vi "Scope_5782_PID.vi"() -> ()   [LabVIEW 2013]
uses:
  <vilib>/userdefined/High Color/nirio_resource_hc.ctl
  FPGA/DataMode.ctl
  <vilib>/Analysis/4window.llb/windowTd.ctl
  Host/Scope/controls/power_spectrum_unit.ctl
  Host/Scope5782/Scope/controls/5782_trigger_type.ctl
  Host/Scope/controls/Data_calc_mode.ctl
  Host/Scope/controls/Data_display_mode.ctl
  Host/Scope/controls/Graph_references.ctl
  Host/Scope/controls/graph_controls.ctl
  Host/Scope/controls/Channel_select.ctl
  Host/Scope5782/Config/FPGAref_5782.ctl
  Host/Communication/response.ctl
  Host/Communication/driver_status.ctl
  Host/Communication/Driver/RemoteConnection/RemoteReferences.ctl
  Host/Communication/Driver/TcpServerDriver/TcpServerDriver.lvclass
  Host/Scope/controls/ScopeMode.ctl
  Host/Communication/global_stop.vi
  <vilib>/FPGAPlugInAG/PXIe-7975R/niLvFpga_Open_PXIe-7975R.vi
  <vilib>/rvi/interface/common/dynamic/niFpgaDynamicAddResources.vi
  <vilib>/rvi/interface/common/niFpgaWaitOnOcc.vi
  <vilib>/Utility/error.llb/Error Cluster From Error Code.vi
  <vilib>/rvi/errors/niLvFpgaAdjustHostInterfaceError.vi
  <vilib>/FPGAPlugInAG/Dynamic/niLvFpga_Close_Dynamic.vi
  <vilib>/rvi/interface/nirviOpenFPGA/nirviOpenFPGA.xnode
  FPGA Bitfiles/mixer_FPGATarget2_FPGAmain5782PIDt_FQeTUQzgJng.lvbitx
  <vilib>/rvi/interface/nirviReadWriteControl/nirviReadWriteControl.xnode
  <vilib>/rvi/interface/nirviCloseFPGA/nirviCloseFPGA.xnode
  Host/Utilities/Ticker/Ticker.lvclass
  NiFpgaLv.dll
  <vilib>/rvi/interface/Simulation/niFpgaSimulationCallBeginRW.vi
  Host/Communication/Driver/RemoteConnection/RemoteConnection.lvclass
  <vilib>/Analysis/NI_AALPro.lvlib
panel:
  in  "Kp":fxp<+/-,32,4>
  in  "Kd/T":fxp<+/-,32,4>
  in  "Ki*T":fxp<+/-,32,4>
  in  "Feedback":bool
  in  "b":fxp<+/-,16,2>
  in  "a":fxp<+/-,16,2>
  in  "Fequency [kHz]":dbl format="%#_8g"
  in  "#bins":i32=1 min=1 max=16
  in  "ch1 DC offset":dbl caption="DC offset\nChannel 1"
  in  "ch0 DC offset":dbl caption="DC offset\nChannel 0"
  in  "Output delay delta":dbl(slide) scale=0.0..6.0
  in  "Output delay":dbl(slide) scale=0.0..6.0
  in  "Chart length":i32=200000
  in  "Trigmode":enum32{"Triggered", "Continuous"}(radio)
  in  "Refence for phase":T1
  in  "Graph_refs":T2
  out "Lower chart":dbl[][](graph)
  out "Upper chart":dbl[][](graph)
  out "Lower graph":i16[][](graph)
  in  "Buffer":T4
  in  "Display":T5
  in  "Output mixer fequency [MHz]":dbl
  in  "Trigger":T6
  in  "Ch1 Q":bool
  in  "Ch1 I":bool
  in  "Ch0 Q":bool
  in  "Ch0 I":bool
  in  "Ch1":bool
  in  "Ch0":bool
  out "stop 2":bool
  in  "Zoom freq X":bool
  in  "Zoom freq Y":bool
  in  "Zoom time Y":bool
  in  "Zoom time X":bool
  in  "Unit":T7
  in  "Window":T8=1 items=["Rectangle"=0, "Hanning"=1, "Hamming"=2, "Blackman-Harris"=3, "Exact Blackman"=4, "Blackman"=5, "Flat Top"=6, "4 Term B-Harris "=7, "7 Term B-Harris"=8, "Low Sidelobe"=9, "Blackman Nuttall"=11, "Triangle"=30, "Bartlett-Hanning"=31, "Bohman"=32, "Parzen"=33, "Welch"=34, "Kaiser"=60, "Dolph-Chebyshev"=61, "Gaussian"=62]
  in  "Samples per 5782 record":i32
  in  "Phase offset (deg)":dbl
  in  "Fequency [MHz]":dbl format="%#_8g"
  in  "Mode":T9
  in  "Mixer freq [MHz]":dbl
  out "freqdata":cluster{"f0":dbl, "df":dbl, "magnitude":dbl[]}[](graph)
  out "Upper graph":i16[][](graph)
  in  "Rumode":bool
  in  "Singleshot":bool
  out "error IO":errorcluster
  in  "stop":bool
  in  "resource name":T10="RIO0"
  out "Clocking Option Configured?":bool
  out "Configured?":bool
  # "FPGA setup"
  # "V"
  # "V"
  # "Output delay"
  # "ns"
  # "Auto Zoom"
  # "Output delay delta"
  # "ps"
  # "5782"
  # "Amplitude modulation"
  # "Simulated data"
  # "FFT"
  # "Auto Zoom"
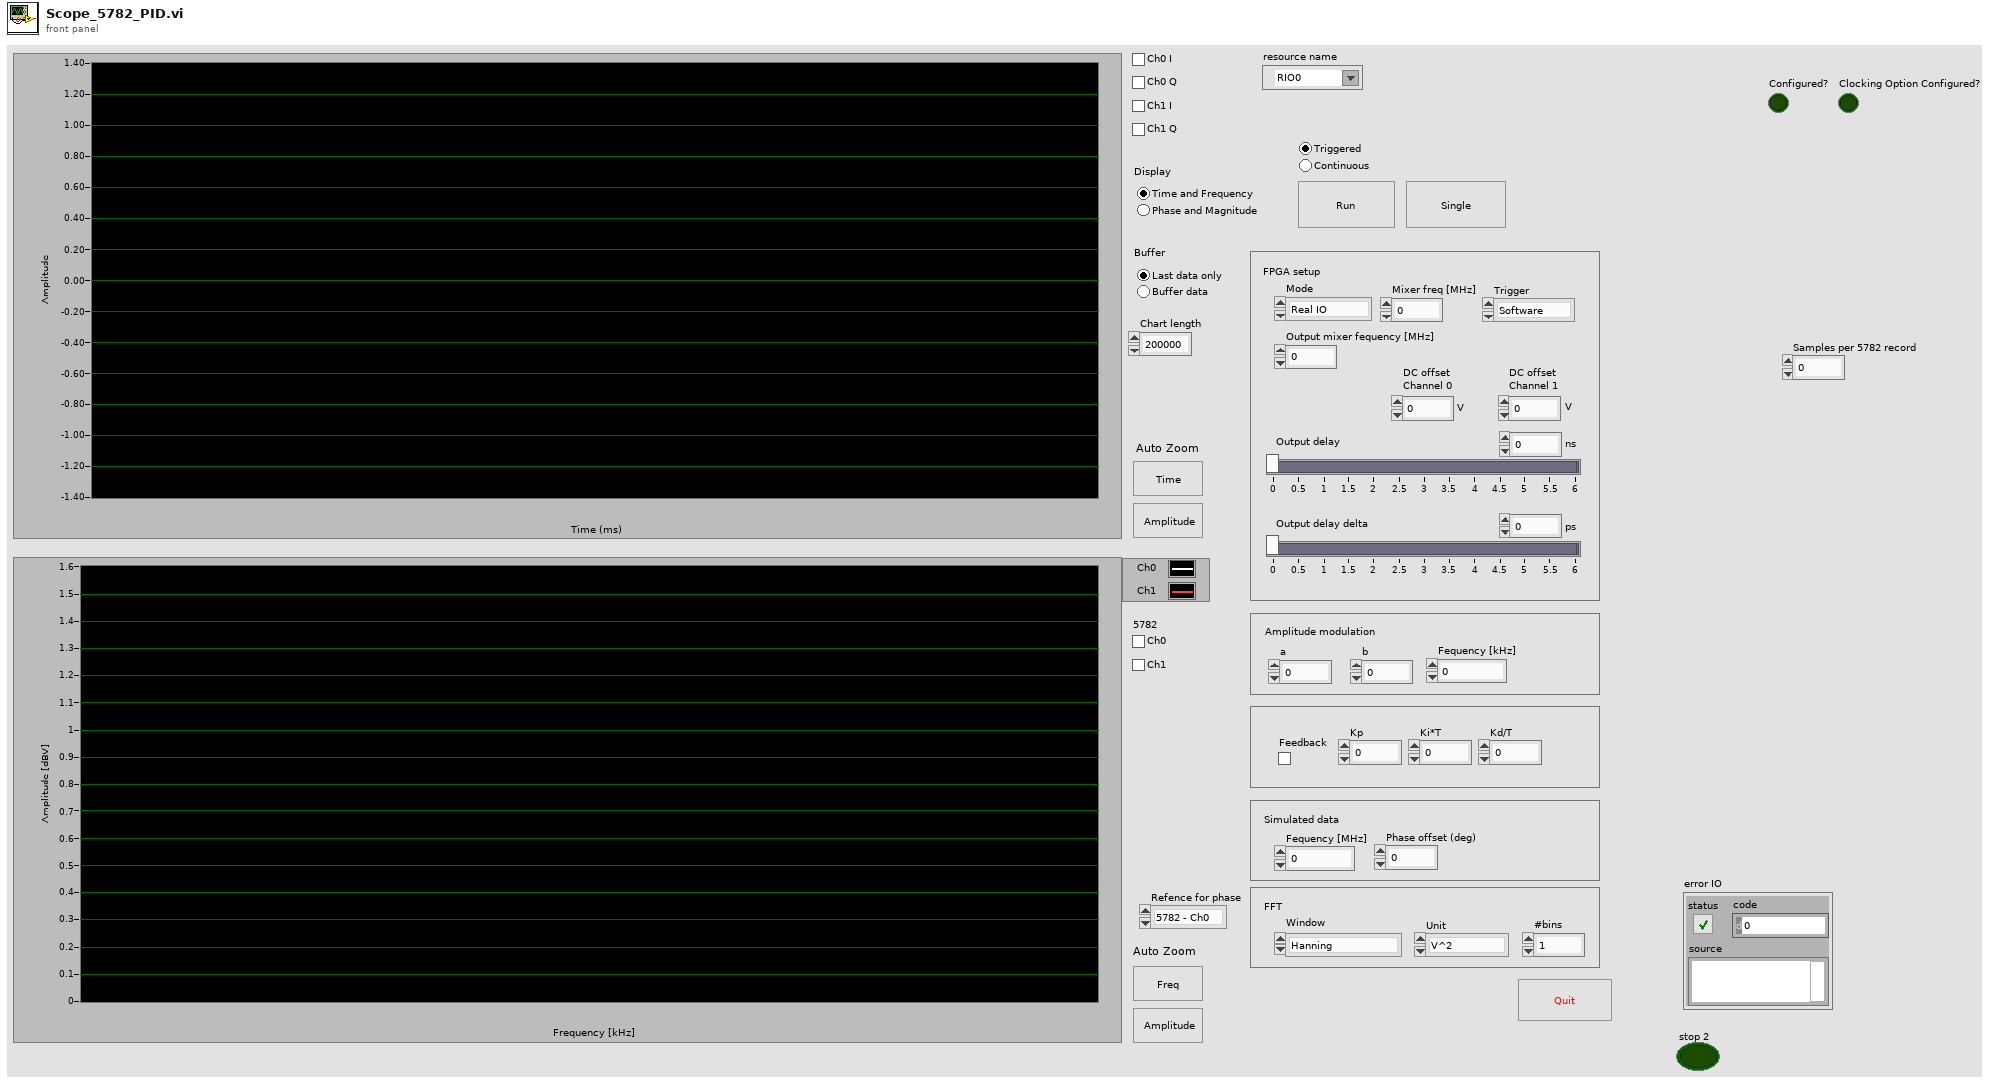
[diagram p1: front panel]
types:
  T1 = typedef "Channel_select.ctl" = enum16{"5782 - Ch0", "5782 - Ch1"}
  T2 = typedef "Graph_references.ctl" = cluster{"upper":T3, "lower":T3, "Freq graph":refnum<vi>}
  T3 = typedef "graph_controls.ctl" = cluster{"Graph":refnum<vi>, "Time btn":refnum<vi>, "Amplitude btn":refnum<vi>, "Chart":refnum<vi>}
  T4 = typedef "Data_display_mode.ctl" = enum32{"Last data only", "Buffer data"}
  T5 = typedef "Data_calc_mode.ctl" = enum32{"Time and Frequency", "Phase and Magnitude"}
  T6 = typedef "5782_trigger_type.ctl" = enum16{"Software", "Trigger input"}
  T7 = typedef "power_spectrum_unit.ctl" = enum16{"V^2", "V", "dBV"}
  T8 = typedef "NI_AALPro.lvlib/windowTd.ctl" = u32
  T9 = typedef "DataMode.ctl" = enum16{"Real IO", "Simulated"}
  T10 = typedef "nirio_resource_hc.ctl" = tag
  T11 = typedef "RemoteConnection.lvclass/RemoteReferences.ctl" = cluster{"a":refnum<vi>, "b":refnum<vi>, "fm":refnum<vi>}
  T12 = typedef "response.ctl" = cluster{"driver status":T13, "Sender":string, "Type":i32, "Variant":variant}
  T13 = typedef "driver_status.ctl" = enum16{"Normal", "Startup", "Connection lost", "Reconnected", "Timeout", "Idle", "Busy"}
  T14 = typedef "FPGAref_5782.ctl" = refnum<k20>
  T15 = enum8{"Internal Clock PLL Off", "Internal Clock PLL On (REF IN)", "External Clock (CLK_IN)", "Internal Clock PLL On (IoModSyncClk)"}
  T16 = typedef "message_queue.ctl" = refnum<queue>
  T17 = typedef "scope_params_5782.ctl" = cluster{"scope mode":T18, "ticker":refnum<class "Ticker.lvclass">, "samples per record":i32, "FPGA ref":T14, "data mode":T9, "5782 Trigger":T6, "Chart length":i32, "RemoteConnection":refnum<class "RemoteConnection.lvclass">}
  T18 = typedef "ScopeMode.ctl" = enum16{"Stopped", "Single", "Running", "Continuous"}
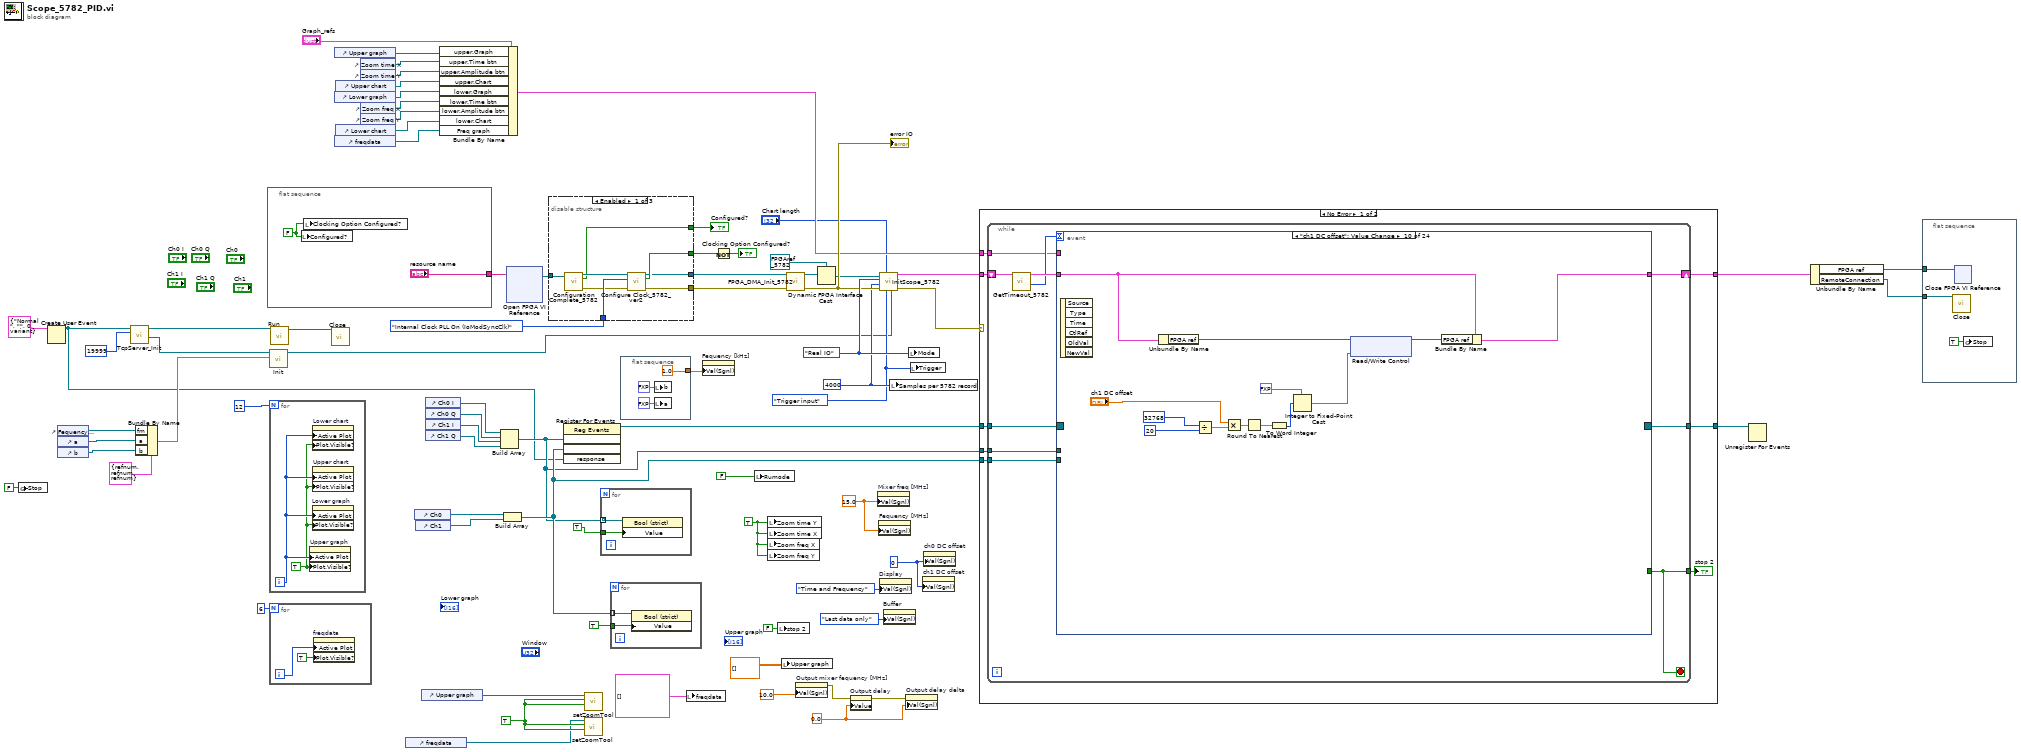
[diagram p0: block diagram]
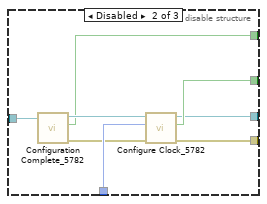
[diagram p2: hidden frame]
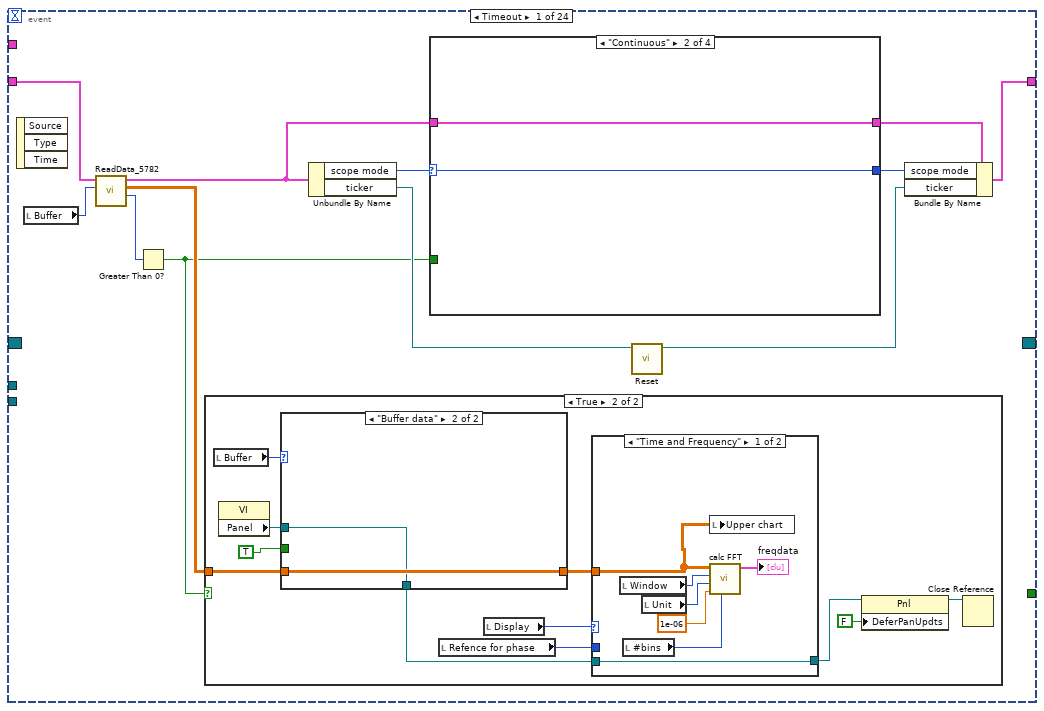
[diagram p4: hidden frame]
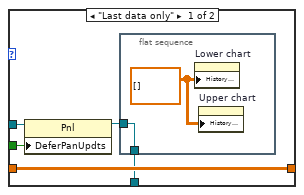
[diagram p6: hidden frame]
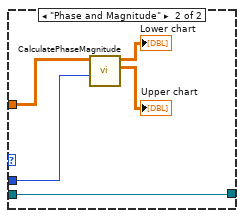
[diagram p7: hidden frame]
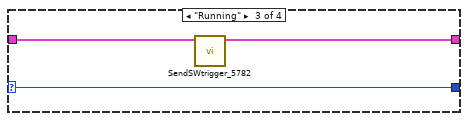
[diagram p9: hidden frame]
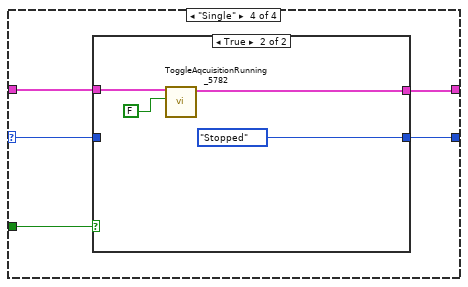
[diagram p10: hidden frame]
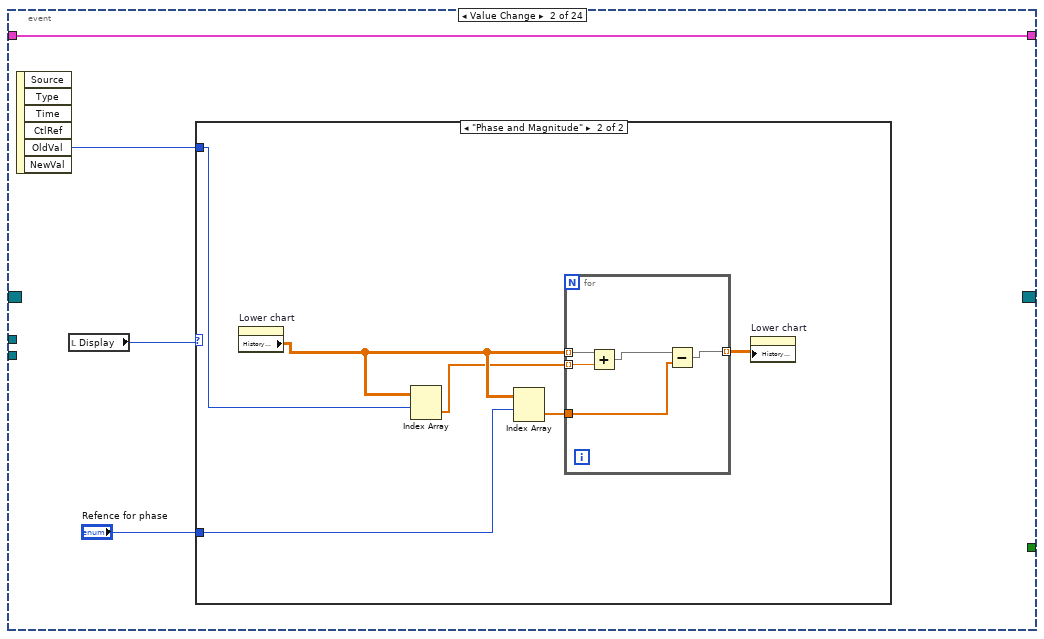
[diagram p12: hidden frame]
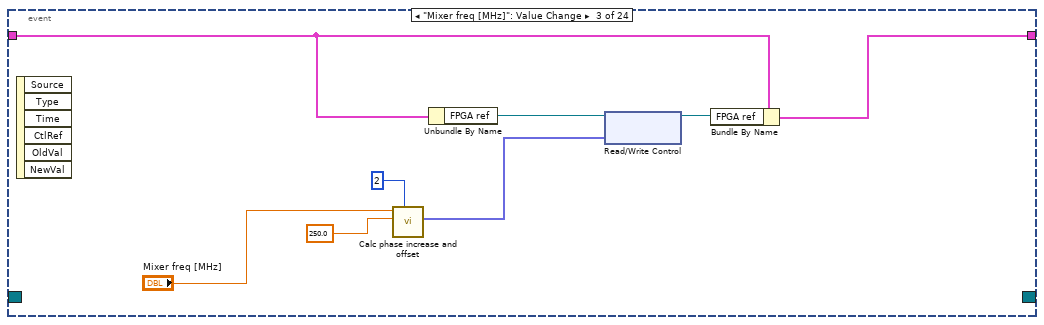
[diagram p14: hidden frame]
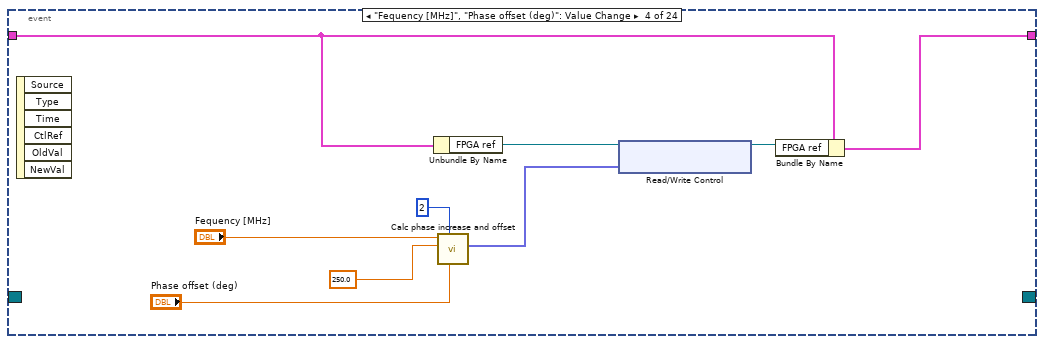
[diagram p15: hidden frame]
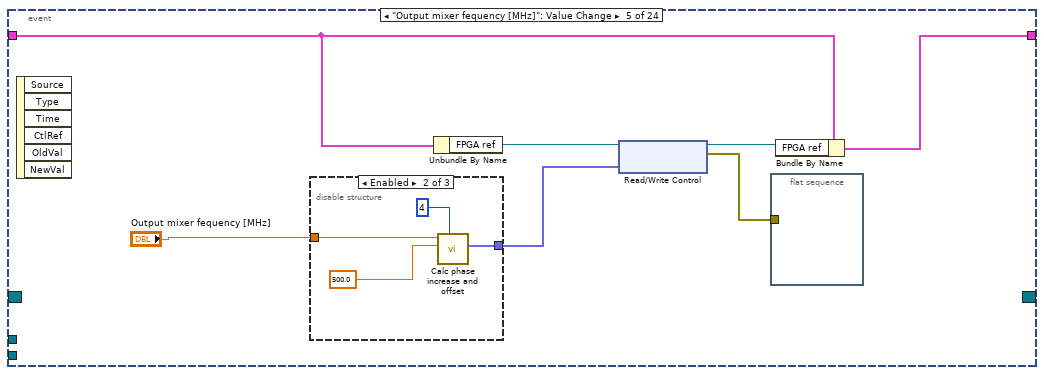
[diagram p16: hidden frame]
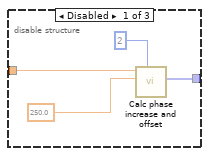
[diagram p17: hidden frame]
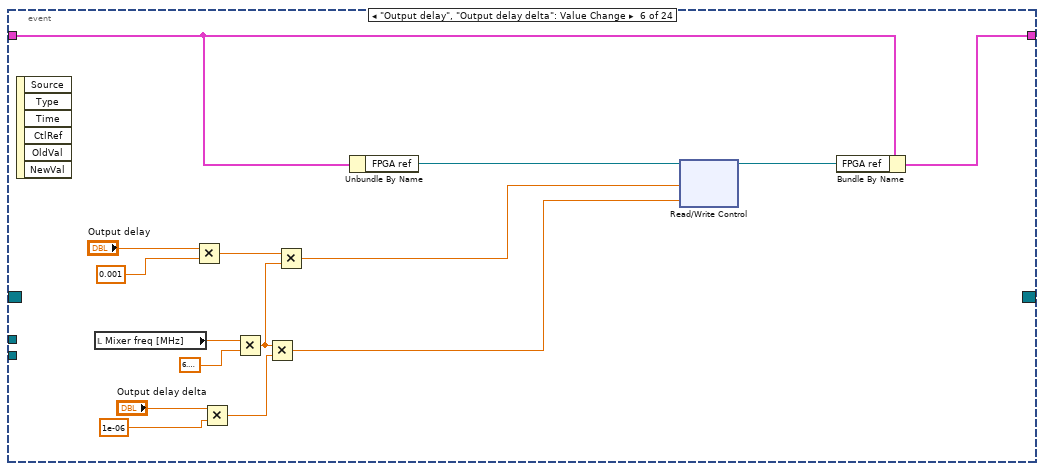
[diagram p19: hidden frame]
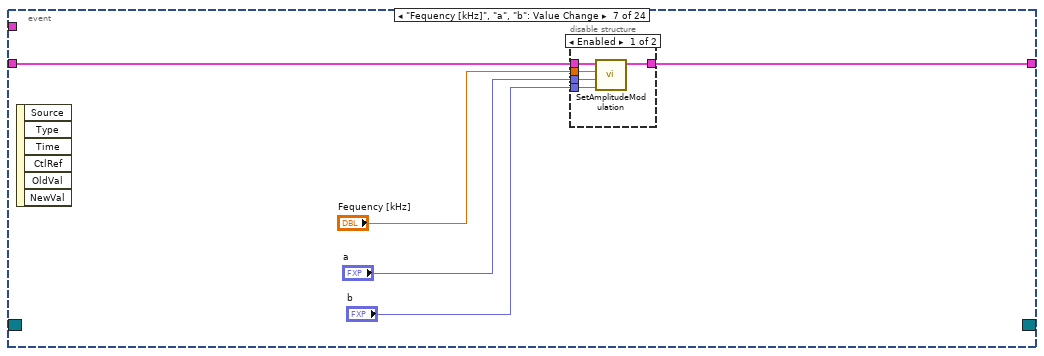
[diagram p20: hidden frame]
diagram:
  w21 = i16 0 ("Value (Signaling)")
  w22 = 0.0 ("Value (Signaling)")
  w45 = 5782_trigger_type."Trigger input" ("Trigger")
  w51 = TRUE ("Zoom  X")
  w61 = TRUE ("Rumode")
  w60 = DataMode."Real IO" ("Mode")
  w47 = 4000 ("Samples to aqcuire")
  w72 = 15.0 ("Mixer requency [MHz]")
  n1 = global write "global_stop.vi" "Stop"(FALSE ("Stop")) -> ()
  n2 = Create User Event(user event datatype=T12 {"driver status"=enum."Normal", "Sender"="", "Type"=0, "Variant"=variant} ("response")) -> (user event=w5:refnum<user-event>)  [unwired: 1 in, 1 out]
  n3 = control-ref of="Fequency [kHz]"() -> (w7:refnum<vi>)
  n4 = control-ref of="a"() -> (w8:refnum<vi>)
  n5 = control-ref of="b"() -> (w6:refnum<vi>)
  n6 = call "TcpServer_Init.vi"("local port"=u16 19999, "response event"=w5) -> ("Message queue"=w13:T16, "TcpServerDriver"=w10:refnum<class "TcpServerDriver.lvclass">)  [unwired: 8 in]
  n7 = Bundle By Name(cluster=T11 {"a"=refnum, "b"=refnum, "fm"=refnum} ("refs"), "fm"=w7, "a"=w8, "b"=w6) -> (w15:T11)
  n8 = flat-sequence {
    tunnel: ["resource name"] -> w62
    frame #0 {
      w77 = FALSE ("Trigger Acquisition")
      n9 = local write "Configured?"(w77) -> ()
      n10 = local write "Clocking Option Configured?"(w77) -> ()
    }
  }
  n11 = call "Init.vi"("refs"=w15, "server queue"=w13) -> ("RemoteConnection"=w4:refnum<class "RemoteConnection.lvclass">)  [unwired: 9 in]
  n12 = for {
    N: 12 -> [_]
    i -> [w80]
    w79 = TRUE ("Plot.Visible")
    n13 = property on="Upper graph" class="WFGraph (strict)"("Active Plot"=w80, "Plot.Visible?"=w79) -> ()  [unwired: 2 in, 2 out]
    n14 = property on="Lower graph" class="WFGraph (strict)"("Active Plot"=w80, "Plot.Visible?"=w79) -> ()  [unwired: 2 in, 2 out]
    n15 = property on="Lower chart" class="WFChart (strict)"("Active Plot"=w80, "Plot.Visible?"=w79) -> ()  [unwired: 2 in, 2 out]
    n16 = property on="Upper chart" class="WFChart (strict)"("Active Plot"=w80, "Plot.Visible?"=w79) -> ()  [unwired: 2 in, 2 out]
  }
  n17 = for {
    N: 6 -> [_]
    i -> [w81]
    n18 = property on="freqdata" class="WFGraph (strict)"("Active Plot"=w81, "Plot.Visible?"=TRUE ("Plot.Visible")) -> ()  [unwired: 2 in, 2 out]
  }
  n19 = call-dynamic "Run.vi"("BaseDriver in"=w10) -> ("BaseDriver out"=w11:refnum<class "TcpServerDriver.lvclass">)  [unwired: 9 in, 1 out]
  n20 = call-dynamic "Close.vi"("BaseDriver in"=w11) -> ()  [unwired: 9 in, 2 out]
  n21 = control-ref of="Upper graph"() -> (w42:refnum<vi>)
  n22 = control-ref of="Lower graph"() -> (w38:refnum<vi>)
  n23 = control-ref of="freqdata"() -> (w34:refnum<vi>)
  n24 = control-ref of="Upper chart"() -> (w39:refnum<vi>)
  n25 = control-ref of="Lower chart"() -> (w35:refnum<vi>)
  n26 = control-ref of="Zoom time X"() -> (w41:refnum<vi>)
  n27 = control-ref of="Zoom time Y"() -> (w40:refnum<vi>)
  n28 = control-ref of="Zoom freq X"() -> (w37:refnum<vi>)
  n29 = control-ref of="Zoom freq Y"() -> (w36:refnum<vi>)
  n30 = control-ref of="freqdata"() -> (w49:refnum<vi>)
  n31 = control-ref of="Ch0"() -> (w57:refnum<vi>)
  n32 = control-ref of="Ch1"() -> (w58:refnum<vi>)
  n33 = control-ref of="Upper graph"() -> (w50:refnum<vi>)
  n34 = control-ref of="Ch0 I"() -> (w53:refnum<vi>)
  n35 = control-ref of="Ch0 Q"() -> (w54:refnum<vi>)
  n36 = control-ref of="Ch1 I"() -> (w55:refnum<vi>)
  n37 = control-ref of="Ch1 Q"() -> (w56:refnum<vi>)
  n38 = Bundle By Name(cluster="Graph_refs", "upper.Graph"=w42, "upper.Time btn"=w41, "upper.Amplitude btn"=w40, "upper.Chart"=w39, "lower.Graph"=w38, "lower.Time btn"=w37, "lower.Amplitude btn"=w36, "lower.Chart"=w35, "Freq graph"=w34) -> (w33:T2)
  n39 = Build Array(w53, w54, w55, w56) -> (w52:refnum<vi>[])
  n40 = Build Array(w57, w58) -> (w64:refnum<vi>[])
  n41 = xnode "Open FPGA VI Reference"("resource name"=w62) -> ("FPGA VI Reference Out"=w27:refnum<k20>)  [unwired: 1 in, 1 out]
  n42 = disable-structure shown="Enabled" {
    disable-tunnel: [w90 w98 _] -> w29
    disable-tunnel: T15."Internal Clock PLL On (IoModSyncClk)" ("Clock Source") -> [w89 w97 _]
    disable-tunnel: [w87 w95 _] -> w28
    disable-tunnel: [w85 w92 w99] -> w20
    disable-tunnel: w27 -> [w83 w94 w99]
    disable-tunnel: [w84 w91 _] -> w25
    frame Enabled {
      n43 = call "Configuration Complete_5782.vi"("FPGA VI Reference in"=w83) -> ("error out"=w88:errorcluster, "Configured?"=w84:bool, "FPGA VI Reference out"=w86:refnum<k20>)  [unwired: 8 in]
      n44 = call "Configure Clock_5782_ver2.vi"("error in"=w88, "Clock Source"=w89, "FPGA VI Reference"=w86) -> ("error out"=w87:errorcluster, "Configuration Error"=w90:bool, "FPGA VI Reference out"=w85:refnum<k20>)  [unwired: 6 in]
    }
    frame Disabled {
      n45 = call "Configuration Complete_5782.vi"("FPGA VI Reference in"=w94) -> ("error out"=w96:errorcluster, "Configured?"=w91:bool, "FPGA VI Reference out"=w93:refnum<k20>)  [unwired: 8 in]
      n46 = call "Configure Clock_5782.vi"("error in"=w96, "Clock Source"=w97, "FPGA VI Reference in"=w93) -> ("error out"=w95:errorcluster, "Configuration Error"=w98:bool, "FPGA VI Reference Out"=w92:T14)  [unwired: 6 in]
    }
    frame Disabled {
    }
  }
  "Configured?" <- w25
  n47 = register-events(w52, w64, w5) -> (reference out=w68:refnum<event-registration>)  [unwired: 2 in, 1 out]
  n48 = call "setZoomTool.vi"("Zoom Y"=w51, "Zoom  X"=w51, "reference"=w49) -> ()  [unwired: 9 in]
  n49 = call "setZoomTool.vi"("Zoom Y"=w51, "Zoom  X"=w51, "reference"=w50) -> ()  [unwired: 9 in]
  n50 = for {
    tunnel: w52 -> [w101] mode=indexing
    tunnel: TRUE ("Rumode") -> [w100]
    n51 = property class="Bool (strict)"(reference=w101, "Value"=w100) -> ()  [unwired: 1 in, 2 out]
  }
  n52 = for {
    tunnel: w64 -> [w103] mode=indexing
    tunnel: TRUE ("Rumode") -> [w102]
    n53 = property class="Bool (strict)"(reference=w103, "Value"=w102) -> ()  [unwired: 1 in, 2 out]
  }
  n54 = flat-sequence {
    tunnel: [1.0 ("Value (Signaling)")] -> w19
    frame #0 {
      n55 = local write "b"(fxp<+/-,16,2> 0.0 ("b")) -> ()
      n56 = local write "a"(fxp<+/-,16,2> 1.0 ("a")) -> ()
    }
  }
  n57 = local write "freqdata"(cluster{"f0":dbl, "df":dbl, "magnitude":dbl[]}[] [] ("freqdata")) -> ()
  n58 = property on="Fequency [kHz]" class="DigNum (strict)"("Val(Sgnl)"=w19) -> ()  [unwired: 2 in, 2 out]
  n59 = Not(x=w29) -> (.not. x?=→"Clocking Option Configured?":bool)
  n60 = local write "Rumode"(FALSE ("Rumode")) -> ()
  n61 = local write "Zoom time Y"(w61) -> ()
  n62 = local write "Zoom time X"(w61) -> ()
  n63 = local write "Zoom freq X"(w61) -> ()
  n64 = local write "Zoom freq Y"(w61) -> ()
  n65 = local write "stop 2"(FALSE ("stop 2")) -> ()
  n66 = local write "Upper graph"(dbl[][] [] ("Timedata")) -> ()
  n67 = call "FPGA_DMA_Init_5782.vi"("error in (no error)"=w28, "FPGA VI Reference"=w20) -> ("error out"=w48:errorcluster, "FPGA VI Out"=w18:refnum<k20>)  [unwired: 7 in, 1 out]
  "error IO" <- w48
  n68 = property on="Output mixer fequency [MHz]" class="DigNum (strict)"("Val(Sgnl)"=10.0 ("Mixer requency [MHz]")) -> (error out=w23:errorcluster)  [unwired: 2 in, 1 out]
  n69 = Dynamic FPGA Interface Cast(Session In=T14 refnum ("FPGA ref"), Type=w18) -> (Session Out=w17:T14)
  n70 = property on="Output delay" class="Slide (strict)"(error in=w23, "Value"=w22) -> (error out=w24:errorcluster)  [unwired: 1 in, 1 out]
  n71 = property on="Mixer freq [MHz]" class="DigNum (strict)"("Val(Sgnl)"=w72) -> ()  [unwired: 2 in, 2 out]
  n72 = property on="Fequency [MHz]" class="DigNum (strict)"("Val(Sgnl)"=w72) -> ()  [unwired: 2 in, 2 out]
  n73 = call "InitScope_5782.vi"("RemoteConnection"=w4, "Trigger"=w45, "Chart length"="Chart length", "error in"=w48, "Samples Per Trigger"=w47, "data mode"=w60, "FPGA ref"=w17) -> ("error out"=w1:errorcluster, "scope params"=w76:T17)  [unwired: 3 in]
  n74 = property on="Display" class="RadioBtnsControl (strict)"("Val(Sgnl)"=Data_calc_mode."Time and Frequency" ("Value (Signaling)")) -> ()  [unwired: 2 in, 2 out]
  n75 = property on="Buffer" class="RadioBtnsControl (strict)"("Val(Sgnl)"=enum32{"Last data only", "Buffer data"}."Last data only" ("Value (Signaling)")) -> ()  [unwired: 2 in, 2 out]
  n76 = local write "Samples per 5782 record"(w47) -> ()
  n77 = property on="Output delay delta" class="Slide (strict)"(error in=w24, "Val(Sgnl)"=w22) -> ()  [unwired: 1 in, 2 out]
  n78 = local write "Mode"(w60) -> ()
  n79 = local write "Trigger"(w45) -> ()
  n80 = property on="ch1 DC offset" class="DigNum (strict)"("Val(Sgnl)"=w21) -> ()  [unwired: 2 in, 2 out]
  n81 = property on="ch0 DC offset" class="DigNum (strict)"("Val(Sgnl)"=w21) -> ()  [unwired: 2 in, 2 out]
  n82 = case shown="No Error" w1 {
    tunnel: w76 -> [w114 w397]
    tunnel: [w113 w397] -> w46
    tunnel: w68 -> [w112 w396]
    tunnel: [w111 w396] -> w67
    tunnel: w52 -> [w110 _]
    tunnel: w64 -> [w109 _]
    tunnel: w33 -> [w107 _]
    frame No Error {
      n83 = while {
        shift-right: [w124] -> w113
        shift-left: w114 -> [w123]
        tunnel: w112 -> [w120]
        tunnel: [w119] -> w111
        tunnel: w110 -> [w118]
        tunnel: w109 -> [w117]
        tunnel: [w116] -> w108
        tunnel: w107 -> [w115]
        stop <- w116 stop-if-true
        n84 = call "GetTimeout_5782.vi"("scope in"=w123) -> ("Time left"=w121:i32, "scope out"=w122:T17)  [unwired: 9 in]
        n85 = event shown="[9] \"ch1 DC offset\": Value Change" {
          selector: w120 -> [_ _ _ _ _ _ _ _ _ _ _ _ _ _ _ _ _ _ _ _ _ _ _ _]
          dyn-events: [_ _ _ _ _ _ _ _ _ _ _ _ _ _ _ _ _ _ _ _ _ _ _ _] -> w119
          timeout: w121 -> [_ _ _ _ _ _ _ _ _ _ _ _ _ _ _ _ _ _ _ _ _ _ _ _]
          tunnel: [_ _ _ _ _ _ _ _ _ _ _ _ _ _ _ _ _ _ "stop" _ _ _ _ _] -> w116
          tunnel: w122 -> [w131 w190 w208 w214 w223 w244 w253 w265 w278 w291 w297 w301 w304 w314 w322 w347 w352 w357 w360 w367 w377 w382 w388 w395]
          tunnel: [w134 w190 w206 w213 w222 w243 w252 w264 w277 w290 w296 w300 w303 w311 w319 w347 w352 w356 w360 w367 w377 w382 w388 w395] -> w124
          tunnel: w118 -> [_ _ _ _ _ _ _ _ _ _ _ _ _ _ _ w346 _ _ _ _ _ _ _ _]
          tunnel: w117 -> [_ _ _ _ _ _ _ _ _ _ _ _ _ _ _ _ w350 _ _ _ _ _ _ _]
          tunnel: w115 -> [_ _ _ _ _ _ _ _ _ _ _ _ _ _ _ _ _ _ _ _ _ _ _ w392]
          event Timeout {
            n86 = event-data() -> ()  [unwired: 1 in, 3 out]
            n87 = local read "Buffer"() -> (w125:T4)
            n88 = call "ReadData_5782.vi"("Buffer mode"=w125, "scope params"=w131) -> ("Num elements"=w127:i32, "data"=w128:dbl[][], "scope params out"=w130:T17)  [unwired: 7 in]
            n89 = Greater Than 0?(x=w127) -> (x > 0?=w126:bool)
            n90 = case shown="True" w126 {
              tunnel: w128 -> [_ w144]
              frame False {
              }
              frame True {
                n91 = local read "Buffer"() -> (w146:T4)
                n92 = property class="VI"() -> ("Panel"=w139:refnum<vi>)  [unwired: 2 in, 2 out]
                n93 = case shown="\"Buffer data\"" w146 {
                  tunnel: w144 -> [w152 w156]
                  tunnel: [w152 w156] -> w145
                  tunnel: w139 -> [w151 w155]
                  tunnel: TRUE ("Defer Panel Updates") -> [w149 _]
                  tunnel: [w148 w155] -> w137
                  frame "Last data only" {
                    n94 = property class="Pnl"(reference=w151, "DeferPanUpdts"=w149) -> (reference out=w150:refnum<vi>)  [unwired: 1 in, 1 out]
                    n95 = flat-sequence {
                      tunnel: w150 -> [w153]
                      tunnel: [w153] -> w148
                      frame #0 {
                        w154 = dbl[][] [] ("History Data")
                        n96 = property on="Lower chart" class="WFChart (strict)"("History Data"=w154) -> ()  [unwired: 2 in, 2 out]
                        n97 = property on="Upper chart" class="WFChart (strict)"("History Data"=w154) -> ()  [unwired: 2 in, 2 out]
                      }
                    }
                  }
                  frame "Buffer data" {
                  }
                }
                n98 = local read "Refence for phase"() -> (w143:T1)
                n99 = local read "Display"() -> (w147:T5)
                n100 = case shown="\"Time and Frequency\"" w147 {
                  tunnel: w145 -> [w159 w168]
                  tunnel: w143 -> [_ w165]
                  tunnel: [w158 w164] -> w141
                  tunnel: w137 -> [w158 w164]
                  frame "Time and Frequency" {
                    n101 = local read "Window"() -> (w160:T8)
                    n102 = local read "#bins"() -> (w157:i32)
                    n103 = local read "Unit"() -> (w161:T7)
                    n104 = local write "Upper chart"(w159) -> ()
                    n105 = call "calc FFT.vi"("#bins"=w157, "dt"=1e-06, "Unit"=w161, "Window"=w160, "data"=w159) -> ("Power Spectrum / PSD"=→"freqdata":cluster{"f0":dbl, "df":dbl, "magnitude":dbl[]}[])  [unwired: 6 in]
                  }
                  frame "Phase and Magnitude" {
                    n106 = call "CalculatePhaseMagnitude.vi"("phase reference channel"=w165, "data"=w168) -> ("Magnitude"=→"Upper chart":dbl[][], "Phase"=→"Lower chart":dbl[][])  [unwired: 8 in]
                  }
                }
                n107 = property class="Pnl"(reference=w141, "DeferPanUpdts"=FALSE ("Defer Panel Updates")) -> (reference out=w140:refnum<vi>)  [unwired: 1 in, 1 out]
                n108 = Close Reference(reference=w140) -> ()  [unwired: 1 in, 1 out]
              }
            }
            n109 = Unbundle By Name(w130) -> ("scope mode"=w133:T18, "ticker"=w136:refnum<class "Ticker.lvclass">)
            n110 = case shown="\"Continuous\"" w133 {
              selector: w133 -> [w170 w172 w175 w176]
              tunnel: [w170 w172 w175 w180] -> w132
              tunnel: w130 -> [w169 w171 w174 w178]
              tunnel: [w169 w171 w173 w177] -> w129
              tunnel: w126 -> [_ _ _ w179]
              frame "Stopped" {
              }
              frame "Continuous" {
              }
              frame "Running" {
                n111 = call "SendSWtrigger_5782.vi"("scope in"=w174) -> ("scope out"=w173:T17)  [unwired: 9 in, 1 out]
              }
              frame "Single" {
                n112 = case shown="True" w179 {
                  tunnel: [w181 ScopeMode."Stopped" ("scope mode")] -> w180
                  tunnel: w178 -> [w182 w185]
                  tunnel: [w182 w184] -> w177
                  tunnel: w176 -> [w181 _]
                  frame False {
                  }
                  frame True {
                    n113 = call "ToggleAqcuisitionRunning_5782.vi"("Acquisition running"=FALSE, "scope in"=w185) -> ("scope out"=w184:T17)  [unwired: 8 in, 1 out]
                  }
                }
              }
            }
            n114 = call "Reset.vi"("Ticker in"=w136) -> ("Ticker out"=w135:refnum<class "Ticker.lvclass">)  [unwired: 9 in, 1 out]
            n115 = Bundle By Name(cluster=w129, "scope mode"=w132, "ticker"=w135) -> (w134:T17)
          }
          event Value Change {
            n116 = event-data() -> ("OldVal"=w187:T1)  [unwired: 1 in, 5 out]
            n117 = local read "Display"() -> (w188:T5)
            n118 = case shown="\"Phase and Magnitude\"" w188 {
              tunnel: "Refence for phase" -> [_ w195]
              tunnel: w187 -> [_ w193]
              frame "Time and Frequency", Default {
              }
              frame "Phase and Magnitude" {
                n119 = property on="Lower chart" class="WFChart (strict)"() -> ("History Data"=w194:dbl[][])  [unwired: 2 in, 2 out]
                n120 = Index Array(array=w194, index (row)=w193) -> (element=w192:dbl[])  [unwired: 1 in]
                n121 = Index Array(array=w194, index (row)=w195) -> (element=w196:dbl[])  [unwired: 1 in]
                n122 = for {
                  tunnel: w194 -> [w199] mode=indexing
                  tunnel: w196 -> [w201]
                  tunnel: [w200] -> w191 mode=indexing
                  tunnel: w192 -> [w198] mode=indexing
                  n123 = Add(x=w199, y=w198) -> (x+y=w197:dbl[])
                  n124 = Subtract(x=w197, y=w201) -> (x-y=w200:dbl[])
                }
                n125 = property on="Lower chart" class="WFChart (strict)"("History Data"=w191) -> ()  [unwired: 2 in, 2 out]
              }
            }
          }
          event "Mixer freq [MHz]": Value Change {
            n126 = event-data() -> ()  [unwired: 1 in, 6 out]
            n127 = call "Calc phase increase and offset.vi"("# of DDS"=2, "fclk (MHz)"=250.0 ("fclk (800MHz)"), "f_generated (MHz)"="Mixer freq [MHz]") -> ("Phase out"=w202:fxp<+,64,64>[])  [unwired: 6 in, 2 out]
            n128 = Unbundle By Name(w208) -> ("FPGA ref"=w209:T14)
            n129 = xnode "Read/Write Control"("FPGA VI Reference In"=w209, "Phase 5782"=w202) -> ("FPGA VI Reference Out"=w207:T14)  [unwired: 1 in, 1 out]
            n130 = Bundle By Name(cluster=w208, "FPGA ref"=w207) -> (w206:T17)
          }
          event "Fequency [MHz]", "Phase offset (deg)": Value Change {
            n131 = event-data() -> ()  [unwired: 1 in, 6 out]
            n132 = Unbundle By Name(w214) -> ("FPGA ref"=w216:T14)
            n133 = call "Calc phase increase and offset.vi"("Phase offset (deg)"="Phase offset (deg)", "# of DDS"=2, "fclk (MHz)"=250.0 ("fclk (800MHz)"), "f_generated (MHz)"="Fequency [MHz]") -> ("Phase out"=w210:fxp<+,64,64>[])  [unwired: 5 in, 2 out]
            n134 = xnode "Read/Write Control"("FPGA VI Reference In"=w216, "Simulated phase 5782"=w210) -> ("FPGA VI Reference Out"=w215:T14)  [unwired: 1 in, 1 out]
            n135 = Bundle By Name(cluster=w214, "FPGA ref"=w215) -> (w213:T17)
          }
          event "Output mixer fequency [MHz]": Value Change {
            n136 = event-data() -> ()  [unwired: 1 in, 6 out]
            n137 = disable-structure shown="Enabled" {
              disable-tunnel: [w227 w231 _] -> w219
              disable-tunnel: "Output mixer fequency [MHz]" -> [w226 w230 _]
              frame Disabled {
                n138 = call "Calc phase increase and offset.vi"("# of DDS"=2, "fclk (MHz)"=250.0 ("fclk (800MHz)"), "f_generated (MHz)"=w226) -> ("Phase out"=w227:fxp<+,64,64>[])  [unwired: 6 in, 2 out]
              }
              frame Enabled {
                n139 = call "Calc phase increase and offset.vi"("# of DDS"=4, "fclk (MHz)"=500.0 ("fclk (800MHz)"), "f_generated (MHz)"=w230) -> ("Phase out"=w231:fxp<+,64,64>[])  [unwired: 6 in, 2 out]
              }
              frame Disabled {
              }
            }
            n140 = Unbundle By Name(w223) -> ("FPGA ref"=w225:T14)
            n141 = xnode "Read/Write Control"("FPGA VI Reference In"=w225, "Phase output"=w219) -> ("FPGA VI Reference Out"=w224:T14, "error out"=w220:errorcluster)  [unwired: 1 in]
            n142 = flat-sequence {
              tunnel: w220 -> [_]
              frame #0 {
              }
            }
            n143 = Bundle By Name(cluster=w223, "FPGA ref"=w224) -> (w222:T17)
          }
          event "Output delay", "Output delay delta": Value Change {
            n144 = event-data() -> ()  [unwired: 1 in, 6 out]
            n145 = local read "Mixer freq [MHz]"() -> (w238:dbl)
            n146 = Multiply(x="Output delay", y=0.001) -> (x*y=w239:dbl)
            n147 = Multiply(x="Output delay delta", y=1e-06) -> (x*y=w241:dbl)
            n148 = Multiply(x=w238, y=6.283185307179586) -> (x*y=w234:dbl)
            n149 = Multiply(x=w234, y=w241) -> (x*y=w235:dbl)
            n150 = Multiply(x=w239, y=w234) -> (x*y=w236:dbl)
            n151 = Unbundle By Name(w244) -> ("FPGA ref"=w248:T14)
            n152 = xnode "Read/Write Control"("FPGA VI Reference In"=w248, "Fi_start"=w236, "Fi_delta"=w235) -> ("FPGA VI Reference Out"=w247:T14)  [unwired: 1 in, 1 out]
            n153 = Bundle By Name(cluster=w244, "FPGA ref"=w247) -> (w243:T17)
          }
          event "Fequency [kHz]", "a", "b": Value Change {
            n154 = event-data() -> ()  [unwired: 1 in, 6 out]
            n155 = disable-structure shown="Enabled" {
              disable-tunnel: w253 -> [w258 w259]
              disable-tunnel: [w257 w259] -> w252
              disable-tunnel: "Fequency [kHz]" -> [w256 _]
              disable-tunnel: "a" -> [w255 _]
              disable-tunnel: "b" -> [w254 _]
              frame Enabled {
                n156 = call "SetAmplitudeModulation.vi"("b_am"=w254, "a_am"=w255, "Am freq [kHz]"=w256, "scope in"=w258) -> ("scope out"=w257:T17)  [unwired: 7 in]
              }
              frame Disabled {
              }
            }
          }
          event "Feedback": Value Change {
            n157 = event-data() -> ()  [unwired: 1 in, 6 out]
            n158 = Unbundle By Name(w265) -> ("FPGA ref"=w267:T14)
            n159 = xnode "Read/Write Control"("FPGA VI Reference In"=w267, "feedback enable"="Feedback", "Ki*Tau"="Ki*T", "Kd/Tau"="Kd/T", "Kp"="Kp") -> ("FPGA VI Reference Out"=w266:T14)  [unwired: 1 in, 1 out]
            n160 = Bundle By Name(cluster=w265, "FPGA ref"=w266) -> (w264:T17)
          }
          event "ch0 DC offset": Value Change {
            n161 = event-data() -> ()  [unwired: 1 in, 6 out]
            n162 = Unbundle By Name(w278) -> ("FPGA ref"=w280:T14)
            n163 = Divide(x=32768, y=20) -> (x/y=w274:dbl)
            n164 = Multiply(x="ch0 DC offset", y=w274) -> (x*y=w273:dbl)
            n165 = Round To Nearest(number=w273) -> (nearest integer value=w272:dbl)
            n166 = To Word Integer(number=w272) -> (16bit integer=w271:i16)
            n167 = Integer to Fixed-Point Cast(fixed-point type=fxp<+/-,16,14> 0.0 ("y"), integer=w271) -> (fixed-point=w269:fxp<+/-,16,14>)
            n168 = xnode "Read/Write Control"("FPGA VI Reference In"=w280, "DC offset chan 0"=w269) -> ("FPGA VI Reference Out"=w279:T14)  [unwired: 1 in, 1 out]
            n169 = Bundle By Name(cluster=w278, "FPGA ref"=w279) -> (w277:T17)
          }
          event "ch1 DC offset": Value Change {
            n170 = event-data() -> ()  [unwired: 1 in, 6 out]
            n171 = Unbundle By Name(w291) -> ("FPGA ref"=w293:T14)
            n172 = Divide(x=32768, y=20) -> (x/y=w287:dbl)
            n173 = Multiply(x="ch1 DC offset", y=w287) -> (x*y=w286:dbl)
            n174 = Round To Nearest(number=w286) -> (nearest integer value=w285:dbl)
            n175 = To Word Integer(number=w285) -> (16bit integer=w284:i16)
            n176 = Integer to Fixed-Point Cast(fixed-point type=fxp<+/-,16,14> 0.0 ("y"), integer=w284) -> (fixed-point=w281:fxp<+/-,16,14>)
            n177 = xnode "Read/Write Control"("FPGA VI Reference In"=w293, "DC offset chan 1"=w281) -> ("FPGA VI Reference Out"=w292:T14)  [unwired: 1 in, 1 out]
            n178 = Bundle By Name(cluster=w291, "FPGA ref"=w292) -> (w290:T17)
          }
          event Value Change {
            n179 = event-data() -> ()  [unwired: 1 in, 6 out]
            n180 = Unbundle By Name(w297) -> ("FPGA ref"=w299:T14)
            n181 = property on="Rumode" class="Bool (strict)"("Val(Sgnl)"=FALSE ("Value (Signaling)")) -> ()  [unwired: 2 in, 2 out]
            n182 = xnode "Read/Write Control"("FPGA VI Reference In"=w299, "Mode"="Mode") -> ("FPGA VI Reference Out"=w298:T14)  [unwired: 1 in, 1 out]
            n183 = Bundle By Name(cluster=w297, "FPGA ref"=w298, "data mode"="Mode") -> (w296:T17)
          }
          event Value Change {
            n184 = event-data() -> ()  [unwired: 1 in, 6 out]
            n185 = Bundle By Name(cluster=w301, "5782 Trigger"="Trigger") -> (w300:T17)
          }
          event "Samples per 5782 record": Value Change {
            n186 = event-data() -> ()  [unwired: 1 in, 6 out]
            n187 = Unbundle By Name(w304) -> ("FPGA ref"=w307:T14)
            n188 = xnode "Read/Write Control"("FPGA VI Reference In"=w307, "5782 record length"="Samples per 5782 record") -> ("FPGA VI Reference Out"=w306:T14)  [unwired: 1 in, 1 out]
            n189 = Bundle By Name(cluster=w304, "FPGA ref"=w306, "samples per record"="Samples per 5782 record") -> (w303:T17)
          }
          event "Singleshot": Value Change {
            n190 = event-data() -> ()  [unwired: 1 in, 6 out]
            n191 = local write "Rumode"(FALSE ("Rumode")) -> ()
            n192 = Bundle By Name(cluster=w314, "scope mode"=ScopeMode."Single") -> (w309:T17)
            n193 = call "ToggleContinousMode.vi"("Cont Acquisition"=FALSE, "scope in"=w309) -> ("scope out"=w308:T17)  [unwired: 8 in, 1 out]
            n194 = call "ToggleAqcuisitionRunning_5782.vi"("Acquisition running"=TRUE, "scope in"=w308) -> ("scope out"=w312:T17)  [unwired: 8 in, 1 out]
            n195 = call "SendSWtrigger_5782.vi"("scope in"=w312) -> ("scope out"=w311:T17)  [unwired: 9 in, 1 out]
          }
          event "Rumode": Value Change {
            n196 = event-data() -> ()  [unwired: 1 in, 6 out]
            n197 = case shown="\"Triggered\"" "Trigmode" {
              tunnel: [ScopeMode."Running" ("scope mode") ScopeMode."Continuous" ("scope mode")] -> w317
              frame "Triggered" {
              }
              frame "Continuous" {
              }
            }
            n198 = Select(t=w317, s="Rumode", f=ScopeMode."Stopped" ("scope mode")) -> (s? t:f=w321:T18)
            n199 = Bundle By Name(cluster=w322, "scope mode"=w321) -> (w320:T17)
            n200 = case shown="\"Single\", \"Running\"" w321 {
              tunnel: w320 -> [w329 w336 w340]
              tunnel: [w330 w334 w341] -> w319
              frame "Single", "Running" {
                n201 = call "ToggleContinousMode.vi"("Cont Acquisition"=FALSE, "scope in"=w329) -> ("scope out"=w327:T17)  [unwired: 8 in, 1 out]
                n202 = call "ToggleAqcuisitionRunning_5782.vi"("Acquisition running"=TRUE, "scope in"=w327) -> ("scope out"=w331:T17)  [unwired: 8 in, 1 out]
                n203 = call "SendSWtrigger_5782.vi"("scope in"=w331) -> ("scope out"=w330:T17)  [unwired: 9 in, 1 out]
              }
              frame "Continuous" {
                n204 = call "ToggleAqcuisitionRunning_5782.vi"("Acquisition running"=TRUE, "scope in"=w336) -> ("scope out"=w335:T17)  [unwired: 8 in, 1 out]
                n205 = call "ToggleContinousMode.vi"("Cont Acquisition"=TRUE ("Acquisition running"), "scope in"=w335) -> ("scope out"=w334:T17)  [unwired: 8 in, 1 out]
              }
              frame "Stopped" {
                n206 = call "ToggleContinousMode.vi"("Cont Acquisition"=FALSE, "scope in"=w340) -> ("scope out"=w338:T17)  [unwired: 8 in, 1 out]
                n207 = call "ToggleAqcuisitionRunning_5782.vi"("Acquisition running"=FALSE, "scope in"=w338) -> ("scope out"=w341:T17)  [unwired: 8 in, 1 out]
              }
            }
          }
          event Value Change {
            n208 = event-data() -> ("CtlRef"=w345:refnum<vi>, "NewVal"=w343:bool)  [unwired: 1 in, 4 out]
            n209 = Search 1D Array(1D array=w346, element=w345) -> (index of element=w344:i32)  [unwired: 1 in]
            n210 = property on="Upper graph" class="WFGraph (strict)"("Active Plot"=w344, "Plot.Visible?"=w343) -> ()  [unwired: 2 in, 2 out]
            n211 = property on="Upper chart" class="WFChart (strict)"("Active Plot"=w344, "Plot.Visible?"=w343) -> ()  [unwired: 2 in, 2 out]
          }
          event Value Change {
            n212 = event-data() -> ("CtlRef"=w351:refnum<vi>, "NewVal"=w348:bool)  [unwired: 1 in, 4 out]
            n213 = Search 1D Array(1D array=w350, element=w351) -> (index of element=w349:i32)  [unwired: 1 in]
            n214 = property on="freqdata" class="WFGraph (strict)"("Active Plot"=w349, "Plot.Visible?"=w348) -> ()  [unwired: 2 in, 2 out]
            n215 = property on="Lower chart" class="WFChart (strict)"("Active Plot"=w349, "Plot.Visible?"=w348) -> ()  [unwired: 2 in, 2 out]
          }
          event User Event {
            n216 = event-data() -> ("Sender"=w355:string, "Variant"=w354:variant, "driver status"=w353:T13)  [unwired: 1 in, 5 out]
            n217 = Unbundle By Name(w357) -> ("RemoteConnection"=w359:refnum<class "RemoteConnection.lvclass">)
            n218 = call "HandleRemoteMessage.vi"("driver status"=w353, "Message data"=w354, "Sender"=w355, "RemoteConnection in"=w359) -> ("RemoteConnection out"=w358:refnum<class "RemoteConnection.lvclass">)  [unwired: 6 in, 1 out]
            n219 = Bundle By Name(cluster=w357, "RemoteConnection"=w358) -> (w356:T17)
          }
          event "stop": Value Change {
            n220 = event-data() -> ()  [unwired: 1 in, 6 out]
          }
          event Value Change {
            n221 = event-data() -> ()  [unwired: 1 in, 6 out]
            n222 = case shown="\"V\"" "Unit" {
              tunnel: ["V" "dBV" "V^2"] -> w364
              frame "V" {
              }
              frame "dBV" {
              }
              frame "V^2" {
              }
            }
            n223 = Concatenate Strings("Amplitude [", w364, "]") -> (w362:string)
            n224 = property on="freqdata" class="WFGraph (strict)"("YScale.NameLbl.Text"=w362) -> ()  [unwired: 2 in, 2 out]
          }
          event "#bins": Value Change {
            n225 = event-data() -> ()  [unwired: 1 in, 6 out]
            n226 = local read "Upper chart"() -> (w373:dbl[][])
            n227 = local read "Window"() -> (w374:T8)
            n228 = local read "Unit"() -> (w375:T7)
            n229 = call "calc FFT.vi"("#bins"="#bins", "dt"=1e-06, "Unit"=w375, "Window"=w374, "data"=w373) -> ("Power Spectrum / PSD"=w372:cluster{"f0":dbl, "df":dbl, "magnitude":dbl[]}[])  [unwired: 6 in]
            n230 = local write "freqdata"(w372) -> ()
          }
          event "Zoom time X", "Zoom time Y": Value Change {
            n231 = event-data() -> ()  [unwired: 1 in, 6 out]
            n232 = control-ref of="Upper chart"() -> (w380:refnum<vi>)
            n233 = control-ref of="Upper graph"() -> (w381:refnum<vi>)
            n234 = call "setZoomTool.vi"("Zoom Y"="Zoom time Y", "Zoom  X"="Zoom time X", "reference"=w380) -> ()  [unwired: 9 in]
            n235 = call "setZoomTool.vi"("Zoom Y"="Zoom time Y", "Zoom  X"="Zoom time X", "reference"=w381) -> ()  [unwired: 9 in]
          }
          event "Zoom freq Y", "Zoom freq X": Value Change {
            n236 = event-data() -> ()  [unwired: 1 in, 6 out]
            n237 = control-ref of="Lower chart"() -> (w386:refnum<vi>)
            n238 = control-ref of="Lower graph"() -> (w385:refnum<vi>)
            n239 = control-ref of="freqdata"() -> (w387:refnum<vi>)
            n240 = call "setZoomTool.vi"("Zoom Y"="Zoom freq Y", "Zoom  X"="Zoom freq X", "reference"=w387) -> ()  [unwired: 9 in]
            n241 = call "setZoomTool.vi"("Zoom Y"="Zoom freq Y", "Zoom  X"="Zoom freq X", "reference"=w386) -> ()  [unwired: 9 in]
            n242 = call "setZoomTool.vi"("Zoom Y"="Zoom freq Y", "Zoom  X"="Zoom freq X", "reference"=w385) -> ()  [unwired: 9 in]
          }
          event Value Change {
            w391 = dbl[][] [] ("History Data")
            n243 = event-data() -> ()  [unwired: 1 in, 6 out]
            n244 = property on="Upper chart" class="WFChart (strict)"("History Data"=w391) -> ()  [unwired: 2 in, 2 out]
            n245 = property on="Lower chart" class="WFChart (strict)"("History Data"=w391) -> ()  [unwired: 2 in, 2 out]
            n246 = local write "freqdata"(cluster{"f0":dbl, "df":dbl, "magnitude":dbl[]}[] [] ("freqdata")) -> ()
            n247 = call "UpdateGraphs.vi"("Buffer mode"="Buffer", "Display mode"="Display", "Graph_refs"=w392) -> ()  [unwired: 9 in]
            n248 = property on="Zoom time X" class="Bool (strict)"("Val(Sgnl)"=TRUE ("Value (Signaling)")) -> ()  [unwired: 2 in, 2 out]
          }
        }
      }
      "stop 2" <- w108
    }
    frame Error {
    }
  }
  n249 = Unregister For Events(event registration refnum=w67) -> ()  [unwired: 1 in, 1 out]
  n250 = Unbundle By Name(w46) -> ("FPGA ref"=w75:T14, "RemoteConnection"=w3:refnum<class "RemoteConnection.lvclass">)
  n251 = flat-sequence {
    tunnel: w75 -> [w400]
    tunnel: w3 -> [w399]
    frame #0 {
      n252 = call "Close.vi"("RemoteConnection in"=w399) -> ()  [unwired: 9 in, 2 out]
      n253 = xnode "Close FPGA VI Reference"("FPGA VI Reference In"=w400) -> ()  [unwired: 1 in, 1 out]
      n254 = global write "global_stop.vi" "Stop"(TRUE ("Stop")) -> ()
    }
  }
